vi "Parser_0xE0_(SubVI).vi"(11 "String in":string) -> (1 "NTelem":i32, 2 "NInt":i32, 3 "NParam":i32)   [LabVIEW 2017, in "LV_Unicorn.lvlib"]
uses:
  LV_Unicorn.lvlib
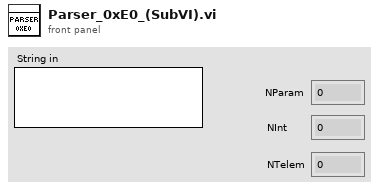
[diagram p1: front panel]
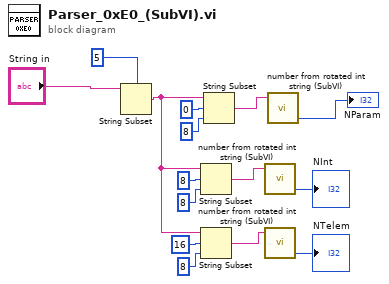
[diagram p0: block diagram]
diagram:
  n1 = String Subset(string="String in", offset (0)=5) -> (substring=w4:string)  [unwired: 1 in]
  n2 = String Subset(string=w4, offset (0)=8, length (rest)=8 ("length (rest)")) -> (substring=w9:string)
  n3 = String Subset(string=w4, offset (0)=16, length (rest)=8 ("length (rest)")) -> (substring=w1:string)
  n4 = String Subset(string=w4, offset (0)=0, length (rest)=8 ("length (rest)")) -> (substring=w13:string)
  n5 = call "number from rotated int string (SubVI).vi"("String"=w9) -> ("int number"=→"NInt":i32)  [unwired: 2 in, 2 out]
  n6 = call "number from rotated int string (SubVI).vi"("String"=w1) -> ("int number"=→"NTelem":i32)  [unwired: 2 in, 2 out]
  n7 = call "number from rotated int string (SubVI).vi"("String"=w13) -> ("int number"=→"NParam":i32)  [unwired: 2 in, 2 out]
